vi "GUID Lookup.vi"() -> ()   [LabVIEW 2013, in "Protection and Rolling Counter Addon Shared.lvlib"]
doc: "Use this Global VI to access the GUIDs assigned to the page resources of the Custom Device."
uses:
  Protection and Rolling Counter Addon Shared.lvlib
panel:
  in  "Protection Valid Channel Page Name":string="Valid"
  in  "Monitor Page Name":string="Monitor"
  in  "Generate Page Name":string="Generate"
  in  "Protection Valid Channel GUID":string="fd6a7400-7849-4da5-96c3-5ff30bdc4abb"
  in  "Monitor GUID":string="bd95a1eb-bc64-4cab-8426-a747b48c9344"
  in  "Generate GUID":string="fe2c6eb8-6675-4af1-b453-994e8ba14209"
  in  "Enable Disable GUID":string="4733d1e7-fc02-4e27-be4e-9d2e12f6fe6f"
  in  "Custom Device GUID_Disabled":string="ac3d5221-c9c0-44f4-a291-06920e8a9c9a"
  in  "Rolling Counter Value GUID":string="94e87467-031b-484c-a85e-bcbac581524d"
  in  "Protection Value GUID":string="ed369b01-8bb7-4d5d-8463-e4aaa20f9c2b"
  in  "Rolling Counter Value":string="Rolling Counter"
  in  "Protection Value":string="Protection"
  in  "Frame Configuration":string="Frame Configuration Settings"
  in  "Frame Configuration Page Name":string="Frame Configuration"
  in  "Frame Configuration GUID":string="bc0c6957-d4ef-4e45-aa02-83c9b233598c"
  in  "Custom Device GUID":string="4d3156ae-de1b-463a-a86e-31c1bc069b17"
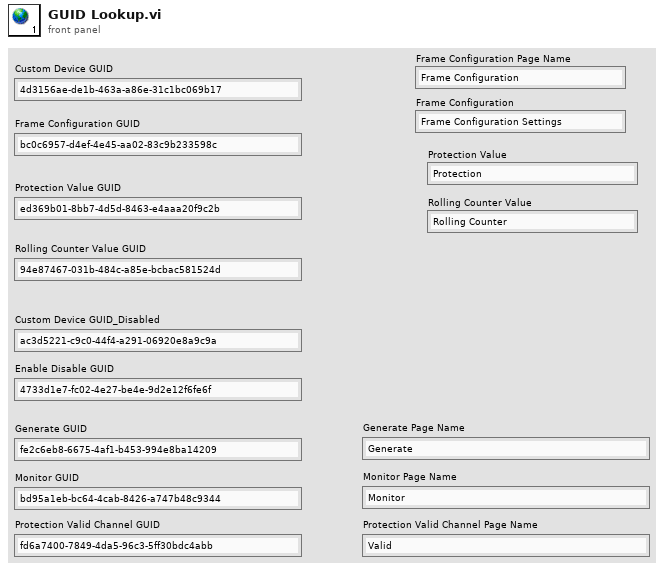
[diagram p1: front panel]
diagram:
